vi "MainInterface_test.vi"() -> ()   [LabVIEW 2018]
uses:
  StateMachine.ctl
  System.Windows.Forms
  <vilib>/Platform/TimedLoop/XDataNode/timing_clust.ctl
  <vilib>/Platform/TimedLoop/XDataNode/nitl_modes.ctl
  <vilib>/Platform/TimedLoop/XDataNode/wakeup.ctl
  <vilib>/platform/TimedLoop/XDataNode/XDataNode.xnode
  General Libraries/Photon Filtering.lvlib
  <vilib>/Platform/TimedLoop/XDataNode/XDNodeRunTimeDep.lvlib
  Read and Save Files/RW_Protocols.lvlib
  General Libraries/myFFT.lvlib
panel:
  in  "PictureBox":refnum<k24>(container)
  out "size(s)":i32[](array[numeric])
  in  "Array":dbl[][](array[numeric])
  out "MemoryGetImageData":variant
  in  "loop state":T1
  out "x > 0?":bool
  out "result array":dbl[][](array[numeric])
  in  "saving name":string="D:\\Data\\Mai\\2019-03-19\\images NbZ=10\\noUS"
  in  "Save all raw images":bool
  in  "run statistics":bool
  in  "flush queue":bool
  in  "Flush Pile":bool
  out "Phase array":dbl[](array[numeric])
  out "sequence NbXZ":dbl[][](array[numeric])
  out "Frame Droped":bool
  in  "buffer":i32
  out "# elements in queue":i32
  in  "Stored data":cluster{dbl, dbl}[](array[cluster])=[{2.048368921229373, 0.13043478260869565}, {2.0513479056383823, 0.2608695652173913}, {2.0543268900473914, 0.043478260869565216}, {2.0573058744564006, 0.08695652173913043}, {2.0602848588654097, 0.34782608695652173}, {2.063263843274419, 0.5217391304347826}, {2.066242827683428, 0.391304347826087}, {2.069221812092437, 0.5652173913043478}, {2.072200796501446, 0.6956521739130435}, {2.0751797809104553, 0.5217391304347826}, {2.0781587653194644, 0.7391304347826086}, {2.0811377497284735, 0.5652173913043478}, {2.0841167341374827, 0.7391304347826086}, {2.087095718546492, 0.5652173913043478}, {2.090074702955501, 0.6086956521739131}, {2.09305368736451, 0.391304347826087}, {2.096032671773519, 0.43478260869565216}, {2.0990116561825283, 0.17391304347826086}, {2.1019906405915374, 0.34782608695652173}, {2.1049696250005465, 0.21739130434782608}, {2.1079486094095556, 0.13043478260869565}, {2.1109275938185648, 0.08695652173913043}, {2.113906578227574, 0.13043478260869565}]
  in  "live":bool
  in  "Tab Control":enum32{"Camera", "Trigger", "configuration"}(tab)
  in  "exposure (us)":i32(slide) caption="exposure" scale=50.0..30000000.0
  in  "gain":i32(slide) scale=32.0..2047.0
  in  "VCD Properties":bool
  in  "Period loop (ms)":i64=150
  in  "sofware triffer":bool
  in  "Trigger ON":bool
  in  "LogFile":bool
  out "error out":errorcluster
  in  "Stop Button":bool
  in  "view tab":T2(tab)
  in  "zoom factor":dbl(slide)=1.0101010101010102 scale=0.0..10.0
  in  "snap FFT":bool
  in  "ICImagingControl":refnum<k7>(container)
  out "Image":T3(plugin-control)
  out "Image Type :":T4 items=["Grayscale (U8)", "Grayscale (I16)", "Grayscale (SGL)", "Complex (CSG)", "RGB (U32)", "HSL (U32)", "RGB (U64)", "Grayscale (U16)"]
  in  "save image 2":bool
  out "data":dbl[][](array[numeric])
  in  "filtered int/phase":bool=TRUE
  in  "Filter on/off":bool=TRUE
  in  "Mask ON":bool
  out "filtered  FFT":dbl[][](graph)
  out "FFT":dbl[][](graph)
  out "value":dbl format="%#_8e"
  in  "Start time":dbl
  in  "FFT int/phase":bool=TRUE
  in  "update loop":bool
  in  "save scan":bool
  out "reconstructed image":dbl[][](graph)
  out "FFT acquire Graph":dbl[][](graph)
  in  "sequence list":i32[](listbox)
  in  "start sequence":bool
  out "N current shoot":i32
  in  "phase offset":dbl format="%#_13g"
  in  "scan name":string="D:\\Data\\Mai\\2019-03-19\\images NbZ=10\\noUS"
  in  "Current scan Tag":i32
  in  "active col":i32
  in  "statistics show":u16(ring)=2 items=["average", "variance", "S/N"]
  out "filtered  averaged":dbl[][](graph)
  out "FFT averaged":dbl[][](graph)
  in  "clear bin":bool
  in  "save noise":bool
  out "Total points num":i32
  out "current averaging":i32
  out "sequence cluster":T5
  out "fft cluster":T6
  # "Watch out more maximum queue size of 200 (update if necessary)"
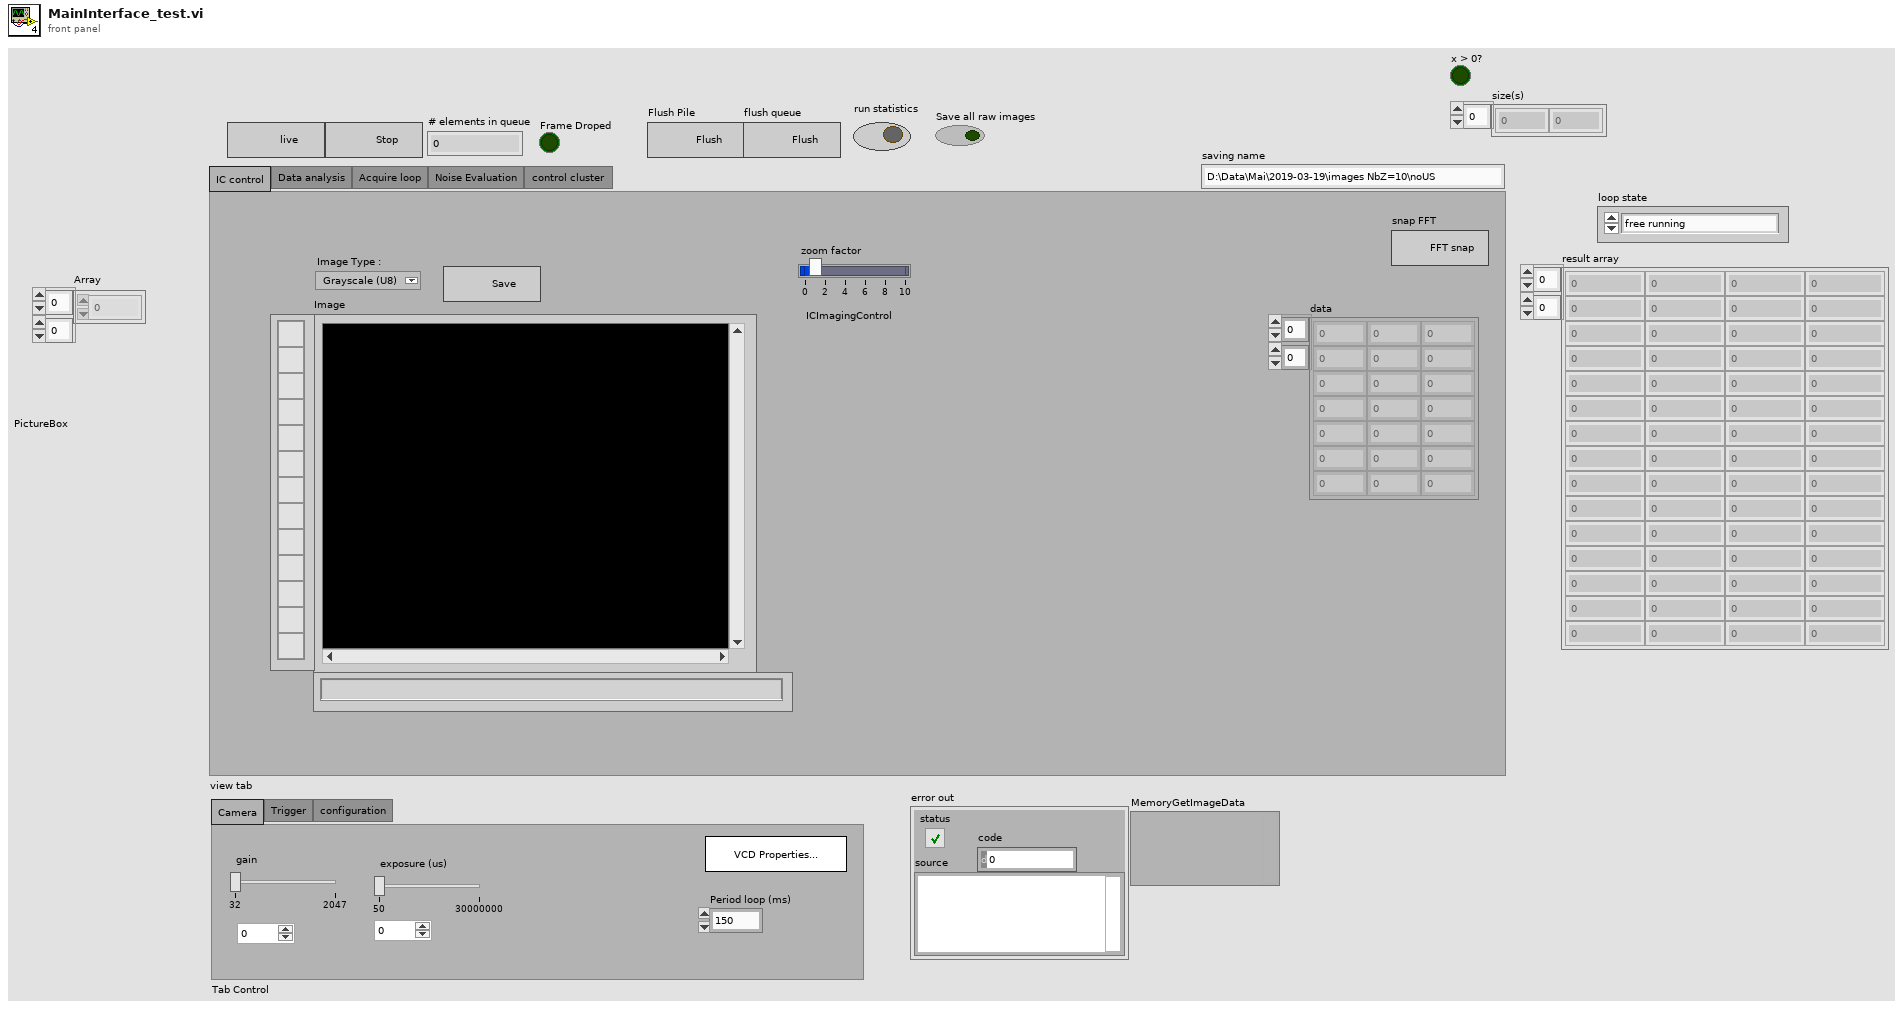
[diagram p1: front panel]
types:
  T1 = typedef "StateMachine.ctl" = enum16{"free running", "sequence recording", "run statistics"}
  T2 = enum32{"IC control", "Data analysis", "Acquire loop", "Noise Evaluation", "control cluster "}
  T3 = typedef "IMAQ Image.ctl" = refnum<image>
  T4 = typedef "Image Type" = u32
  T5 = cluster{"TypeOfSequence":string, "FreqSonde":dbl, "NbHemicycle":dbl, "Tau_cam":dbl, "DurWaveform":dbl, "Prof":dbl, "Nevent":i32, "nuX0":dbl, "nuZ0":dbl}
  T6 = cluster{"dFx":dbl, "dFy":dbl, "Nx":i32, "Ny":i32, "FxMax":dbl, "FyMax":dbl, "Xwidth":dbl, "Ywidth":dbl, "dx":dbl, "dy":dbl, "Fx points":dbl[], "X points":dbl[], "Y points":dbl[], "Fy points":dbl[]}
  T7 = enum8{"Enabled", "Disabled", "Disabled and Grayed Out"}
  T8 = cluster{"Nx fft":i32, "Fx Vector":dbl[], "Ny fft":i32, "Fy-Vector":dbl[]}
  T9 = cluster{"Image Pixels (U16)":u16[][], "Start time":dbl, "buffer":i32}
  T10 = typedef "XDNodeRunTimeDep.lvlib/timing_clust.ctl" = cluster{"Expected End [f-1]":u64, "Actual End [f-1]":u64, "Finished Late? [f-1]":bool, "Expected End [i-1]":u64, "Actual End [i-1]":u64, "Finished Late? [i-1]":bool, "Expected Start [i]":u64, "Actual Start [i]":u64, "Expected Start [f]":u64, "Actual Start [f]":u64, "Source Name":string, "Structure Name":string, "Period":i64, "Deadline":i64, "Offset":i64, "Start":i64, "Priority":i32, "Timeout":i32, "Mode":T11, "Wakeup Reason":T12, "Error":errorcluster, "Source Type":string, "Secondary Source Type":string, "Global End Time":u64, "Global Start Time":u64, "Frame Duration":u64, "Iteration Duration":u64, "Assigned CPU":i32, "I/O Scan Engine Mode":u32}
  T11 = typedef "XDNodeRunTimeDep.lvlib/nitl_modes.ctl" = enum32{"No Change", "Process missed periods, maintain original phase", "Discard missed periods, maintain original phase", "Process missed periods, ignore original phase", "Discard missed periods, ignore original phase"}
  T12 = typedef "XDNodeRunTimeDep.lvlib/wakeup.ctl" = enum32{"Normal", "Aborted", "Asynchronous wakeup", "Timing source error", "Timed loop error", "Timeout"}
  T13 = enum16{"Brightness", "Color Enable", "Contrast", "Exposure", "Focus", "Gain", "Gamma", "Hue", "Iris", "Pan", "Roll", "Saturation", "Sharpness", "Tilt", "Whitebalance", "Zoom", "Whitebalance Blue", "Whitebalance Red"}
  T14 = cluster{"Rows Per Strip":i32, "Photometric":i32, "Compression Type":i32}
  T15 = cluster{"Image Pixels (U16)":u16[][], "SampleStartTime":dbl, "Index":i32}
  T16 = cluster{"Filter on/off":bool, "filtered int/phase":bool, "Mask ON":bool, "FFT int/phase":bool}
  T17 = cluster{"tagged photons":dbl[][], "FFT modulous":dbl[][]}
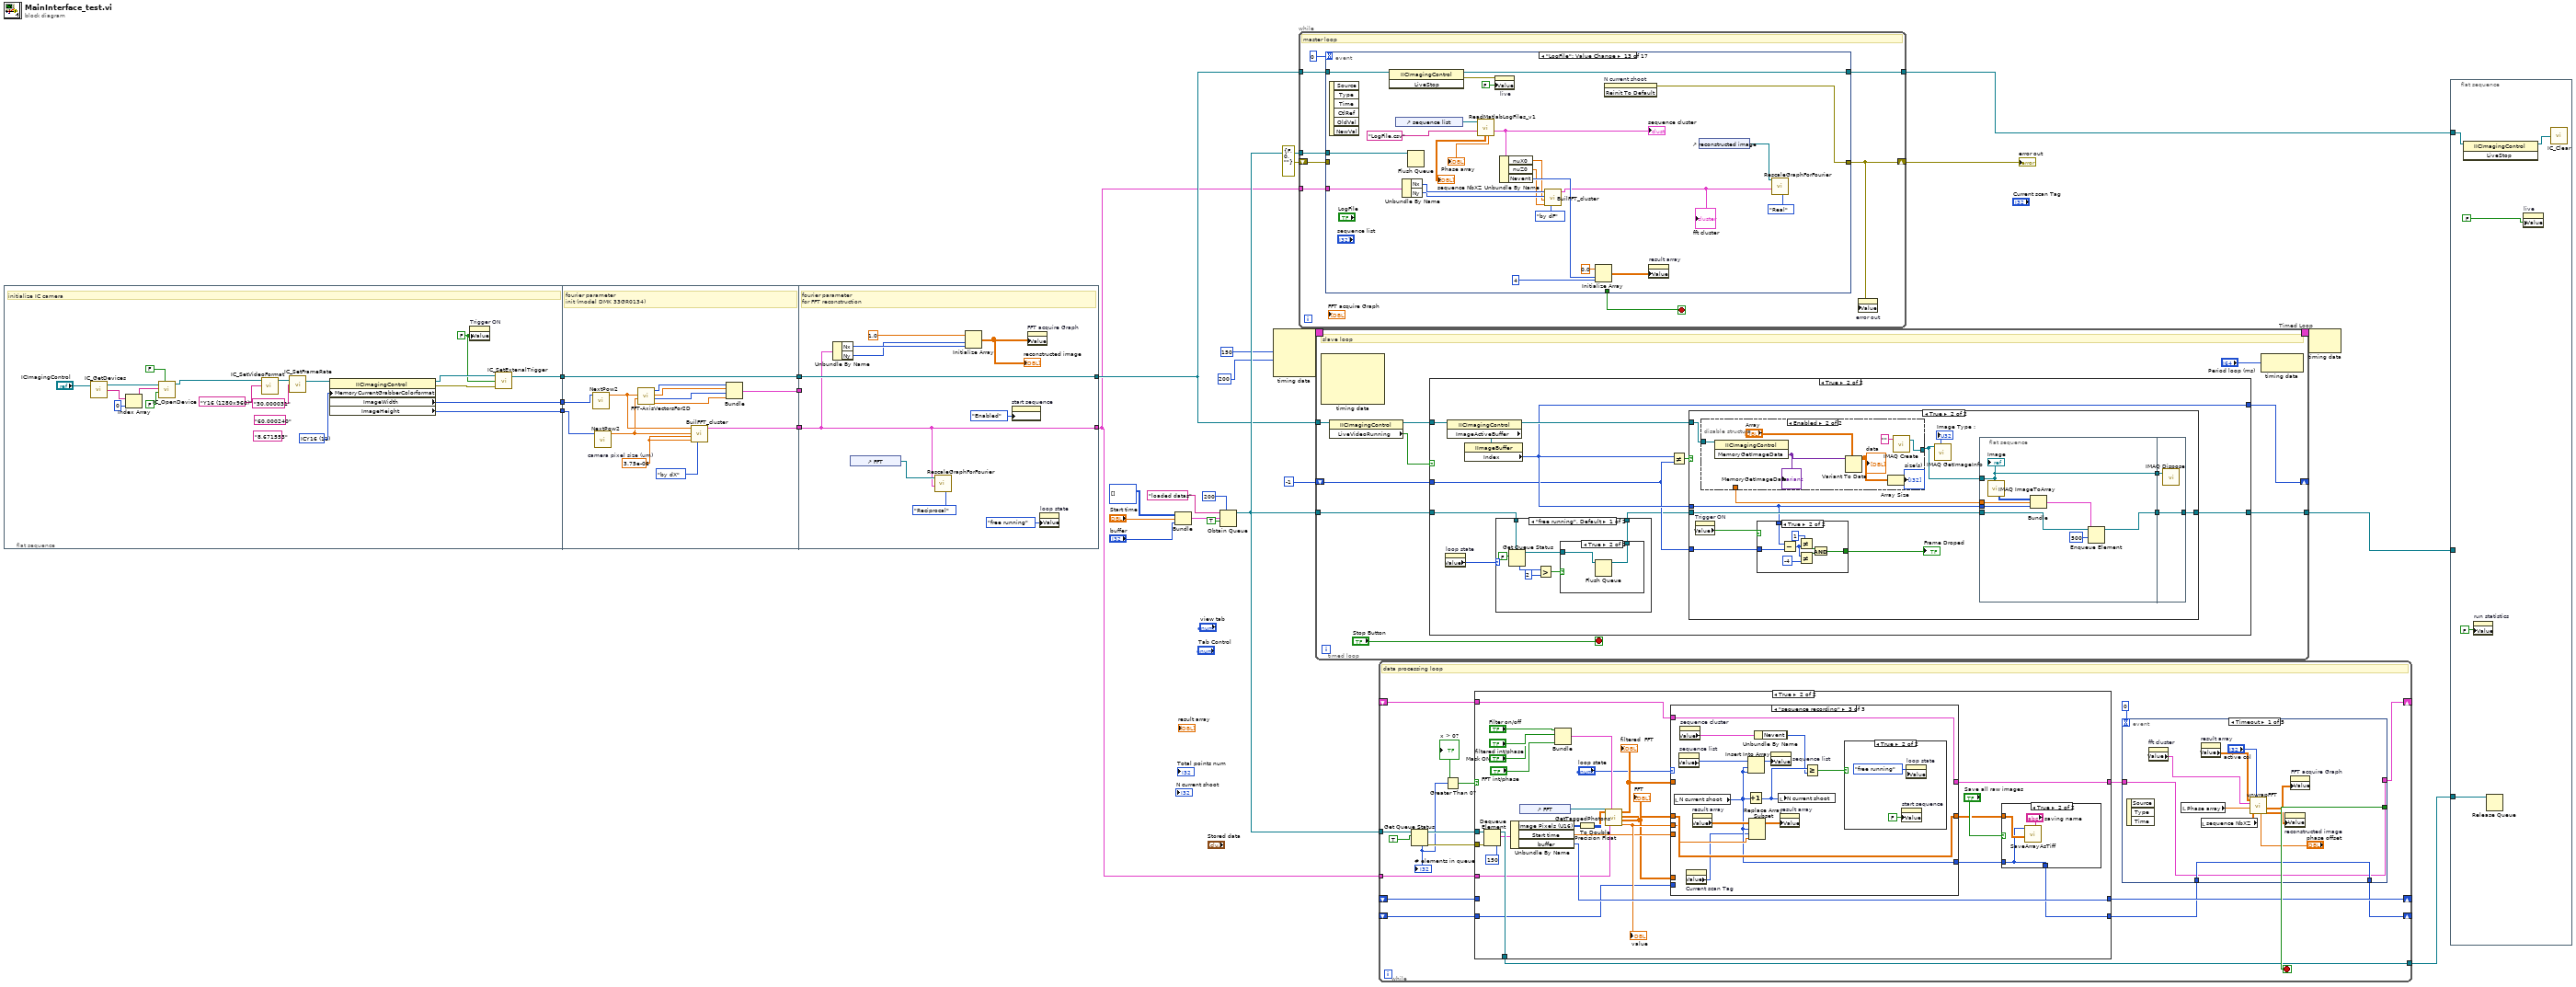
[diagram p0: block diagram]
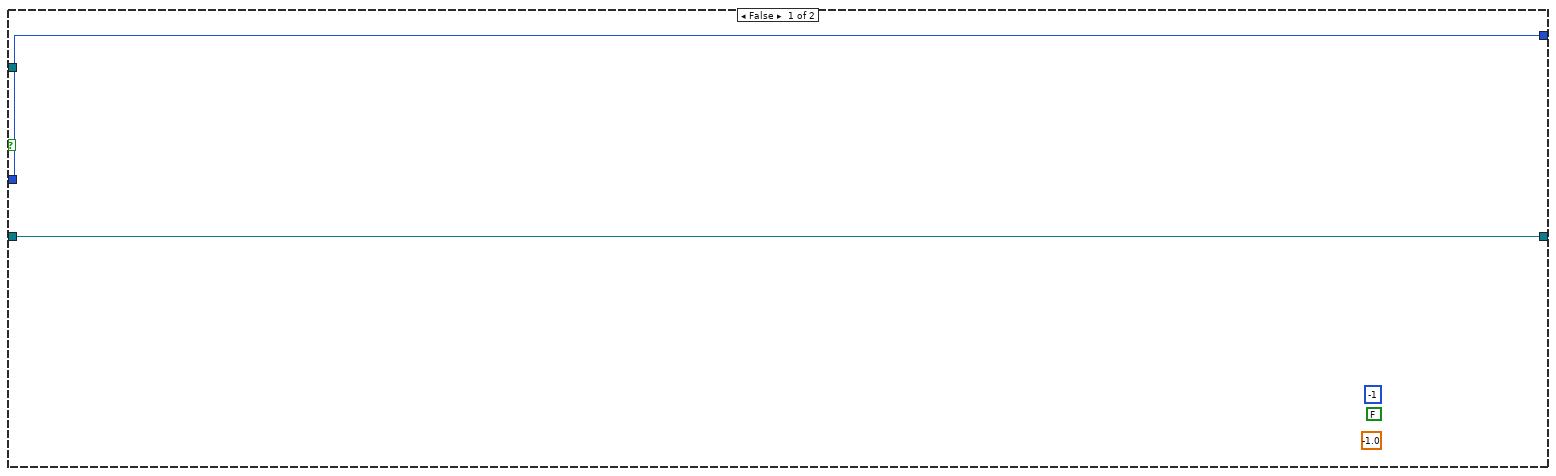
[diagram p2: hidden frame]
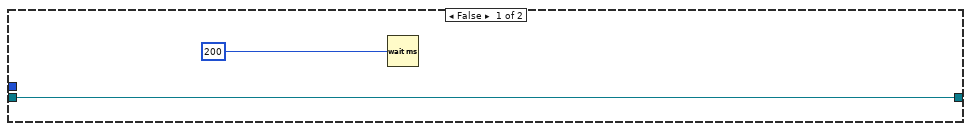
[diagram p5: hidden frame]
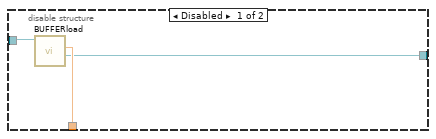
[diagram p6: hidden frame]
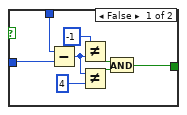
[diagram p7: hidden frame]
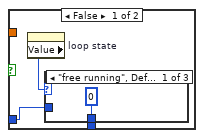
[diagram p9: hidden frame]
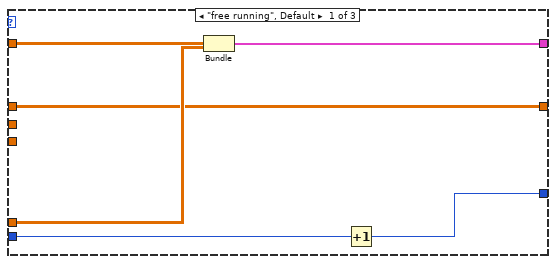
[diagram p12: hidden frame]
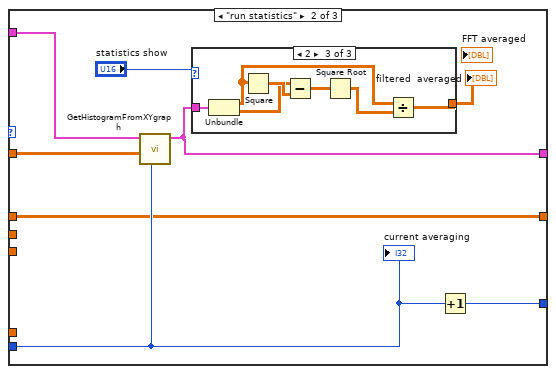
[diagram p13: hidden frame]
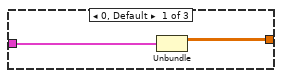
[diagram p14: hidden frame]
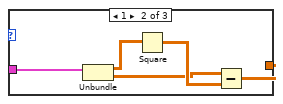
[diagram p15: hidden frame]
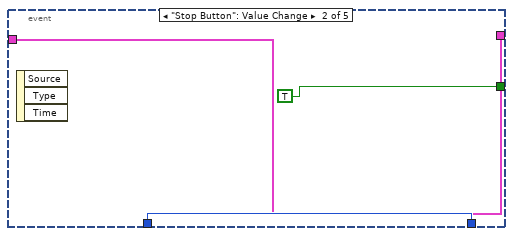
[diagram p17: hidden frame]
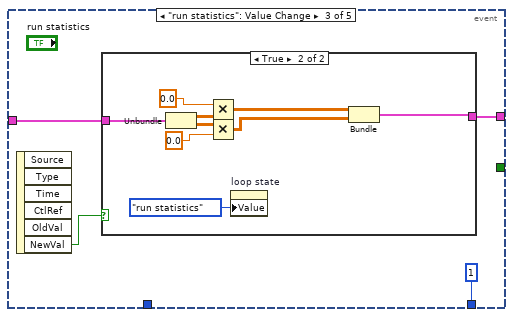
[diagram p18: hidden frame]
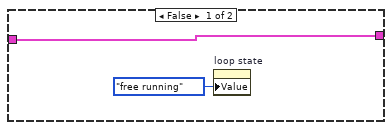
[diagram p19: hidden frame]
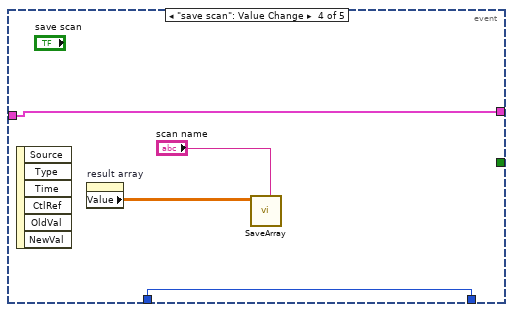
[diagram p20: hidden frame]
diagram:
  n1 = flat-sequence {
    tunnel: [w30] -> w9
    tunnel: [w28] -> w8
    tunnel: [w27] -> w7
    tunnel: w9 -> [w58]
    tunnel: w8 -> [w57]
    tunnel: w7 -> [w56]
    tunnel: [w58] -> w6
    tunnel: [w51] -> w5
    tunnel: [w47] -> w3
    tunnel: [w68] -> w20
    tunnel: w6 -> [w68]
    tunnel: w5 -> [_]
    tunnel: [w60] -> w2
    tunnel: w3 -> [w60]
    frame #0 {
      w31 = FALSE ("Trigger ON")
      (unwired) "8,671553"
      (unwired) "60,000240" ("FrameRate")
      w35 = 11 items=["ICRGB32"=1, "ICRGB24"=2, "ICRGB565"=3, "ICRGB555"=4, "ICY8"=5, "ICUYVY"=6, "ICY800"=7, "ICYGB1"=8, "ICYGB0"=9, "ICBY8"=10, "ICY16"=11] ("MemoryCurrentGrabberColorformat")
      # "initialize IC camera"
      n2 = call <userlib>:"IC_GetDevices.vi"("ICImagingControl In"="ICImagingControl") -> ("ICImagingControl Out"=w42:refnum<k7>, "Devices"=w44:string[])  [unwired: 1 in, 1 out]
      n3 = Index Array(array=w44, index=0) -> (element=w41:string)
      n4 = call <userlib>:"IC_OpenDevice.vi"("Color"=FALSE, "Live"=FALSE, "Device"=w41, "ICImagingControl In"=w42) -> ("ICImagingControl Out"=w38:refnum<k7>)  [unwired: 2 in, 5 out]
      n5 = call <userlib>:"IC_SetVideoFormat.vi"("VideoFormat"="Y16 (1280x960)", "ICImagingControl In"=w38) -> ("ICImagingControl Out"=w37:refnum<k7>)  [unwired: 1 in, 2 out]
      n6 = call <userlib>:"IC_SetFrameRate.vi"("FrameRate"="30,000031", "ICImagingControl In"=w37) -> ("ICImagingControl Out"=w36:refnum<k7>)  [unwired: 1 in, 1 out]
      n7 = property class="IICImagingControl"(reference=w36, "MemoryCurrentGrabberColorformat"=w35) -> (reference out=w32:refnum<k7>, error out=w29:errorcluster, "ImageWidth"=w28:i32, "ImageHeight"=w27:i32)  [unwired: 1 in]
      n8 = property on="Trigger ON" class="Bool (strict)"("Value"=w31) -> ()  [unwired: 2 in, 2 out]
      n9 = call <userlib>:"IC_SetExtenalTrigger.vi"("Error In (no error)"=w29, "Trigger"=w31, "ICImagingControl In"=w32) -> ("ICImagingControl Out"=w30:refnum<k7>)  [unwired: 1 out]
    }
    frame #1 {
      w48 = 3.75e-06  # camera pixel size (um)
      # "fourier parameter\ninit (model DMK 33GR0134)"
      n10 = call "NextPow2.vi"("x"=w57) -> ("2^x"=w50:dbl)  [unwired: 10 in]
      n11 = call "NextPow2.vi"("x"=w56) -> ("2^x"=w49:dbl)  [unwired: 10 in]
      n12 = call "FFT-AxisVectorsFor2D.vi"("Ny in"=w49, "Nx in"=w50) -> ("Fy-Vector"=w52:dbl[], "Ny fft"=w53:i32, "Fx Vector"=w54:dbl[], "Nx fft"=w55:i32)  [unwired: 6 in]
      n13 = call "BuilFFT_cluster.vi"("Enum"=enum16{"by dF", "by dX"}."by dX", "input Y"=w48, "input X"=w48, "Ny"=w49, "Nx"=w50) -> ("fft cluster"=w47:T6)  [unwired: 6 in]
      n14 = Bundle("Nx fft"=w55, "Fx Vector"=w54, "Ny fft"=w53, "Fy-Vector"=w52) -> (w51:T8)  [unwired: 1 in]
    }
    frame #2 {
      # "fourier parameter\nfor FFT reconstruction"
      n15 = Unbundle By Name(w60) -> ("Nx"=w66:i32, "Ny"=w65:i32)
      n16 = control-ref of="FFT"() -> (w62:refnum<vi>)
      n17 = call "RescaleGraphForFourier.vi"("fft reference"=w62, "fft cluster"=w60, "Enum"=enum16{"Reciprocal", "Real"}."Reciprocal") -> ()  [unwired: 8 in]
      n18 = Initialize Array(1.0 ("r"), w65, w66) -> (w64:dbl[][])
      "reconstructed image" <- w64
      n19 = property on="start sequence" class="Bool (strict)"("DisabledEnum"=T7."Enabled" ("Disabled")) -> ()  [unwired: 2 in, 2 out]
      n20 = property on="FFT acquire Graph" class="IntGraph (strict)"("Value"=w64) -> ()  [unwired: 2 in, 2 out]
      n21 = property on="loop state" class="Enum (strict)"("Value"=StateMachine."free running" ("loop state")) -> ()  [unwired: 2 in, 2 out]
    }
  }
  n22 = Bundle("Image Pixels (U16)"=u16[][] [], "Start time"="Start time", "buffer"="buffer") -> (w23:T9)  [unwired: 1 in]
  n23 = Obtain Queue(max queue size (-1, unlimited)=200, name (unnamed)="loaded datas", element data type=w23, create if not found? (T)=TRUE) -> (queue out=w22:refnum<queue>)  [unwired: 1 in, 2 out]
  n24 = node-c288(i64 150 ("Period"), 200 ("Priority")) -> (w15:T10)  [unwired: 2 in]
  n25 = while {
    tunnel: w20 -> [w75]
    tunnel: [w76] -> w16
    shift-right: [w70] -> w17
    shift-left: errorcluster {"status"=FALSE, "code"=0, "source"=""} ("error out") -> [w74]
    tunnel: w22 -> [w73]
    tunnel: w2 -> [w69]
    stop <- w72 stop-if-true
    # "master loop"
    n26 = event shown="[12] \"LogFile\": Value Change" {
      selector: _ -> [_ _ _ _ _ _ _ _ _ _ _ _ _ _ _ _ _]
      dyn-events: _ -> [_ _ _ _ _ _ _ _ _ _ _ _ _ _ _ _ _]
      timeout: 0 -> [_ _ _ _ _ _ _ _ _ _ _ _ _ _ _ _ _]
      tunnel: [_ TRUE _ _ _ _ _ _ _ _ _ _ _ _ _ _ _] -> w72
      tunnel: [w77 w80 _ w84 w86 w97 w102 w105 _ w114 _ w128 w152 w158 w171 w182 w192] -> w76
      tunnel: w75 -> [w77 w80 _ w85 w87 w94 w103 w104 _ w115 w123 w129 w153 w157 w175 w183 w193]
      tunnel: [w78 w79 _ _ w88 w96 w100 w106 _ w113 w125 _ w145 _ _ _ w191] -> w70
      tunnel: w74 -> [w78 w79 w82 _ w88 w95 w101 w107 _ w112 _ _ _ _ _ _ w191]
      tunnel: w73 -> [_ _ w83 _ _ _ _ _ w110 _ _ _ w149 _ _ _ _]
      tunnel: w69 -> [_ _ _ _ _ _ _ _ _ _ _ _ w143 _ _ _ _]
      event Timeout {
        n27 = event-data() -> ()  [unwired: 1 in, 3 out]
      }
      event "Stop Button": Value Change {
        n28 = event-data() -> ()  [unwired: 1 in, 6 out]
      }
      event "flush queue": Value Change {
        n29 = event-data() -> ()  [unwired: 1 in, 6 out]
        n30 = Flush Queue(queue=w83, error in (no error)=w82) -> ()  [unwired: 3 out]
      }
      event "VCD Properties": Value Change {
        n31 = event-data() -> ()  [unwired: 1 in, 6 out]
        n32 = invoke class="IICImagingControl" method="ShowPropertyDialog"(reference=w85) -> (reference out=w84:refnum<k7>)  [unwired: 2 in, 2 out]
      }
      event "live": Value Change {
        n33 = event-data() -> ("NewVal"=w89:bool)  [unwired: 1 in, 5 out]
        n34 = case shown="False" w89 {
          tunnel: w87 -> [w91 w93]
          tunnel: [w90 w92] -> w86
          frame False {
            n35 = invoke class="IICImagingControl" method="LiveStop"(reference=w91) -> (reference out=w90:refnum<k7>)  [unwired: 2 in, 2 out]
          }
          frame True {
            n36 = call <userlib>:"IC_LiveStart.vi"("ICImagingControl 3"=w93) -> ("ICImagingControl 2"=w92:refnum<k7>)
          }
        }
      }
      event "zoom factor": Value Change {
        n37 = event-data() -> ()  [unwired: 1 in, 6 out]
        n38 = property class="IICImagingControl" props=["ZoomRange"](reference=w94, error in=w95) -> (reference out=w97:refnum<k7>, error out=w96:errorcluster)  [unwired: 1 out]
      }
      event "exposure (us)": Value Change {
        n39 = event-data() -> ()  [unwired: 1 in, 6 out]
        n40 = call <userlib>:"IC_SetPropertyValue.vi"("Error In (no error)"=w101, "Value"="exposure (us)", "Property"=T13."Exposure", "ICImagingControl In"=w103) -> ("Error Out"=w100:errorcluster, "ICImagingControl Out"=w102:refnum<k7>)
      }
      event "gain": Value Change {
        n41 = event-data() -> ()  [unwired: 1 in, 6 out]
        n42 = call <userlib>:"IC_SetPropertyValue.vi"("Error In (no error)"=w107, "Value"="gain", "Property"=T13."Gain", "ICImagingControl In"=w104) -> ("Error Out"=w106:errorcluster, "ICImagingControl Out"=w105:refnum<k7>)
      }
      event "Flush Pile": Value Change {
        n43 = event-data() -> ()  [unwired: 1 in, 6 out]
        n44 = Flush Queue(queue=w110) -> ()  [unwired: 1 in, 3 out]
      }
      event "Trigger ON": Value Change {
        n45 = event-data() -> ("NewVal"=w111:bool)  [unwired: 1 in, 5 out]
        n46 = call <userlib>:"IC_SetExtenalTrigger.vi"("Error In (no error)"=w112, "Trigger"=w111, "ICImagingControl In"=w115) -> ("Error Out"=w113:errorcluster, "ICImagingControl Out"=w114:refnum<k7>)
      }
      event "save image 2": Value Change {
        n47 = event-data() -> ()  [unwired: 1 in, 6 out]
        n48 = invoke class="IICImagingControl" method="LiveStop"(reference=w123) -> (reference out=w122:refnum<k7>)  [unwired: 2 in, 2 out]
        n49 = property class="IICImagingControl" props=["ImageActiveBuffer"](reference=w122) -> (reference out=w119:refnum<k7>)  [unwired: 1 in, 2 out]
        n50 = property on="saving name" class="Str"() -> ("Value"=w117:string)  [unwired: 2 in, 2 out]
        n51 = call "FetchTargetFile.vi"("Use default Folder"=TRUE, "FileName"=w117) -> ("Full File Path"=w116:path)  [unwired: 9 in]
        n52 = call "BUFFERload.vi"("ICImagingControl In"=w119) -> ("Image Out"=w120:T3)  [unwired: 6 in, 4 out]
        n53 = call-poly "IMAQ Write File 2"("TIFF Options"=T14 {"Rows Per Strip"=0, "Photometric"=1, "Compression Type"=0}, "File Path"=w116, "Image"=w120) -> ("error out"=w126:errorcluster, "Image Out (duplicate)"=w121:T3)  [unwired: 7 in]
        n54 = call "IMAQ Dispose"("Image"=w121, "error in (no error)"=w126) -> ("error out"=w125:errorcluster)  [unwired: 4 in]
      }
      event "snap FFT": Value Change {
        n55 = event-data() -> ()  [unwired: 1 in, 6 out]
        n56 = invoke class="IICImagingControl" method="LiveStop"(reference=w129) -> (reference out=w131:refnum<k7>)  [unwired: 2 in, 2 out]
        n57 = property class="IICImagingControl" props=["ImageActiveBuffer"](reference=w131) -> (reference out=w130:refnum<k7>)  [unwired: 1 in, 2 out]
        n58 = call <userlib>:"IC_ActiveBuffer_to_IMAQ.vi"("ICImagingControl In"=w130) -> ("ICImagingControl Out"=w128:refnum<k7>, "Image Out"=w127:T3)  [unwired: 2 in, 2 out]
        n59 = call "IMAQ ImageToArray"("Image"=w127) -> ()  [unwired: 3 in, 5 out]
        n60 = call "IMAQ Dispose"() -> ()  [unwired: 6 in, 1 out]
      }
      event "LogFile": Value Change {
        n61 = event-data() -> ()  [unwired: 1 in, 6 out]
        n62 = invoke class="IICImagingControl" method="LiveStop"(reference=w153) -> (reference out=w152:refnum<k7>, error out=w151:errorcluster)  [unwired: 2 in, 1 out]
        n63 = control-ref of="sequence list"() -> (w155:refnum<vi>)
        n64 = Unbundle By Name(w143) -> ("Nx"=w141:i32, "Ny"=w140:i32)
        n65 = Flush Queue(queue=w149) -> ()  [unwired: 1 in, 3 out]
        n66 = call "ReadMatlabLogFiles_v1.vi"("FileName"="LogFile.csv" ("FileName For Matlab load"), "sequence list REF"=w155) -> ("sequence cluster"=w148:T5, "Phase array unit"=→"Phase array":dbl[], "all values"=→"sequence NbXZ":dbl[][])  [unwired: 4 in, 3 out]
        "sequence cluster" <- w148
        n67 = property on="live" class="Bool (strict)"(error in=w151, "Value"=FALSE ("live")) -> ()  [unwired: 1 in, 2 out]
        n68 = Unbundle By Name(w148) -> ("nuX0"=w139:dbl, "nuZ0"=w138:dbl, "Nevent"=w147:i32)
        n69 = call "BuilFFT_cluster.vi"("Enum"=enum16{"by dF", "by dX"}."by dF", "input Y"=w138, "input X"=w139, "Ny"=w140, "Nx"=w141) -> ("fft cluster"=w137:T6)  [unwired: 6 in]
        "fft cluster" <- w137
        n70 = Initialize Array(0.0 ("element"), w147, 4 ("dimension size")) -> (w133:dbl[][])
        n71 = invoke on="N current shoot" class="DigNum (strict)" method="Reinit To Default"() -> (error out=w145:errorcluster)  [unwired: 3 in, 2 out]
        n72 = property on="result array" class="Arr (strict)"("Value"=w133) -> ()  [unwired: 2 in, 2 out]
        n73 = control-ref of="reconstructed image"() -> (w136:refnum<vi>)
        n74 = call "RescaleGraphForFourier.vi"("fft reference"=w136, "fft cluster"=w137, "Enum"=enum16{"Reciprocal", "Real"}."Real") -> ()  [unwired: 8 in]
      }
      event "start sequence": Value Change {
        n75 = event-data() -> ("NewVal"=w156:bool)  [unwired: 1 in, 5 out]
        n76 = case shown="True" w156 {
          tunnel: [w162 w167] -> w158
          tunnel: w157 -> [w163 w166]
          frame False {
            n77 = invoke class="IICImagingControl" method="LiveStop"(reference=w163) -> (reference out=w162:refnum<k7>, error out=w161:errorcluster)  [unwired: 2 in, 1 out]
            n78 = property on="live" class="Bool (strict)"(error in=w161, "Value"=FALSE ("live")) -> ()  [unwired: 1 in, 2 out]
            n79 = property on="loop state" class="Enum (strict)"("Value"=StateMachine."free running" ("loop state")) -> ()  [unwired: 2 in, 2 out]
          }
          frame True {
            n80 = flat-sequence {
              tunnel: w166 -> [w168]
              tunnel: [w168] -> w165
              frame #0 {
                n81 = Wait (ms)(milliseconds to wait=u32 10) -> ()  [unwired: 1 out]
                n82 = property on="loop state" class="Enum (strict)"("Value"=StateMachine."sequence recording" ("loop state")) -> ()  [unwired: 2 in, 2 out]
              }
            }
            n83 = invoke class="IICImagingControl" method="LiveStart"(reference=w165) -> (reference out=w167:refnum<k7>)  [unwired: 2 in, 2 out]
            n84 = property on="live" class="Bool (strict)"("Value"=TRUE ("live")) -> ()  [unwired: 2 in, 2 out]
          }
        }
      }
      event "update loop": Value Change {
        n85 = event-data() -> ()  [unwired: 1 in, 6 out]
        n86 = invoke class="IICImagingControl" method="LiveStop"(reference=w175) -> (reference out=w172:refnum<k7>, error out=w173:errorcluster)  [unwired: 2 in, 1 out]
        n87 = property on="live" class="Bool (strict)"(error in=w173, "Value"=FALSE ("live")) -> ()  [unwired: 1 in, 2 out]
        n88 = flat-sequence {
          tunnel: w172 -> [w180]
          tunnel: [w180] -> w171
          frame #0 {
            n89 = property on="Current scan Tag" class="DigNum (strict)"() -> ("Value"=w178:i32)  [unwired: 2 in, 2 out]
            n90 = property on="sequence list" class="MCListbox (strict)"("Value"=i32[] []) -> ()  [unwired: 2 in, 2 out]
            n91 = Increment(x=w178) -> (x+1=w177:i32)
            n92 = property on="N current shoot" class="DigNum (strict)"("Value"=0 ("N current shoot")) -> ()  [unwired: 2 in, 2 out]
            n93 = property on="Current scan Tag" class="DigNum (strict)"("Value"=w177) -> ()  [unwired: 2 in, 2 out]
          }
        }
      }
      event "clear bin": Value Change {
        n94 = event-data() -> ()  [unwired: 1 in, 6 out]
        n95 = property on="live" class="Bool (strict)"() -> ("Value"=w181:bool)  [unwired: 2 in, 2 out]
        n96 = case shown="True" w181 {
          tunnel: w183 -> [w184 w190]
          tunnel: [w184 w188] -> w182
          frame False {
          }
          frame True {
            n97 = invoke class="IICImagingControl" method="LiveStop"(reference=w190) -> (reference out=w189:refnum<k7>)  [unwired: 2 in, 2 out]
            n98 = property on="Total points num" class="DigNum (strict)"("Value"=0 ("Total points num")) -> (error out=w185:errorcluster)  [unwired: 2 in, 1 out]
            n99 = invoke on="Total points num" class="DigNum (strict)" method="Reinit To Default"(error in=w185) -> (error out=w187:errorcluster)  [unwired: 2 in, 2 out]
            n100 = invoke class="IICImagingControl" method="LiveStart"(reference=w189, error in=w187) -> (reference out=w188:refnum<k7>)  [unwired: 1 in, 2 out]
          }
        }
      }
      event "sofware triffer": Value Change {
        n101 = event-data() -> ()  [unwired: 1 in, 6 out]
        n102 = call <userlib>:"IC_SoftwareTrigger.vi"("ICImagingControl 3"=w193) -> ("ICImagingControl 2"=w192:refnum<k7>)
      }
    }
    n103 = property on="error out" class="Clust (strict)"("Value"=w70) -> ()  [unwired: 2 in, 2 out]
  }
  "error out" <- w17
  n104 = timed-loop "Timed Loop" {
    tunnel: w20 -> [w201]
    shift-right: [w198] -> _
    shift-left: -1 ("Index") -> [w202]
    tunnel: w22 -> [w197]
    tunnel: [w196] -> w19
    timing: w15 -> [_]
    timing-out: [_] -> w14
    stop <- "Stop Button" stop-if-true
    # "slave loop"
    n105 = node-c288() -> ()  [unwired: 1 in, 5 out]
    n106 = property class="IICImagingControl"(reference=w201) -> (reference out=w200:refnum<k7>, "LiveVideoRunning"=w199:bool)  [unwired: 1 in, 1 out]
    n107 = case shown="True" w199 {
      tunnel: w202 -> [w208 w212]
      tunnel: w200 -> [_ w218]
      tunnel: [w208 w213] -> w198
      tunnel: w197 -> [w207 w211]
      tunnel: [w207 w214] -> w196
      frame False {
        (unwired) -1.0 ("SampleStartTime")
        (unwired) FALSE
        (unwired) -1 ("Index")
      }
      frame True {
        n108 = property on="loop state" class="Enum (strict)"() -> ("Value"=w209:T1)  [unwired: 2 in, 2 out]
        n109 = property class="IICImagingControl"(reference=w218) -> (reference out=w216:refnum<k7>, "ImageActiveBuffer"=w217:refnum<k7>)  [unwired: 1 in, 1 out]
        n110 = property class="IImageBuffer"(reference=w217) -> ("Index"=w213:i32)  [unwired: 1 in, 2 out]
        n111 = case shown="\"free running\", Default" w209 {
          tunnel: w211 -> [w225 w229]
          tunnel: [w220 w229] -> w210
          frame "free running", Default {
            n112 = Get Queue Status(queue=w225, return elements? (F)=FALSE) -> (queue out=w221:refnum<queue>, # elements in queue=w224:i32)  [unwired: 1 in, 6 out]
            n113 = Greater?(x=w224, y=2) -> (0:w222:bool)
            n114 = case shown="True" w222 {
              tunnel: w221 -> [w226 w228]
              tunnel: [w226 w227] -> w220
              frame False {
              }
              frame True {
                n115 = Flush Queue(queue=w228) -> (queue out=w227:refnum<queue>)  [unwired: 1 in, 2 out]
              }
            }
          }
          frame "sequence recording" {
          }
        }
        n116 = Not Equal?(x=w213, y=w212) -> (x != y?=w215:bool)
        n117 = case shown="True" w215 {
          tunnel: w216 -> [_ w243]
          tunnel: w210 -> [w230 w242]
          tunnel: [w230 w241] -> w214
          tunnel: w213 -> [_ w234]
          tunnel: w212 -> [_ w235]
          frame False {
            n118 = Wait (ms)(milliseconds to wait=u32 200) -> ()  [unwired: 1 out]
          }
          frame True {
            n119 = property on="Trigger ON" class="Bool (strict)"() -> ("Value"=w232:bool)  [unwired: 2 in, 2 out]
            n120 = disable-structure shown="Enabled" {
              disable-tunnel: w243 -> [w246 w253]
              disable-tunnel: [w245 _] -> w240
              disable-tunnel: [w244 w252] -> w239
              frame Disabled {
                n121 = call "BUFFERload.vi"("ICImagingControl In"=w246) -> ("Image Out"=w244:T3, "SampleStartTime"=w245:dbl)  [unwired: 6 in, 3 out]
              }
              frame Enabled {
                n122 = invoke class="IICImagingControl" method="MemoryGetImageData"(reference=w253) -> ("MemoryGetImageData"=w249:variant)  [unwired: 2 in, 2 out]
                "MemoryGetImageData" <- w249
                n123 = Variant To Data(type="Array", Variant=w249) -> (data=w248:dbl[][])  [unwired: 1 in, 1 out]
                "data" <- w248
                n124 = Array Size(array=w248) -> (size(s)=→"size(s)":i32[])
                n125 = call "IMAQ Create"("Image Name"="") -> ("New Image"=w252:T3)  [unwired: 4 in, 1 out]
              }
            }
            n126 = case shown="True" w232 {
              tunnel: w235 -> [w257 w266]
              tunnel: w234 -> [w256 w265]
              tunnel: [w255 w262] -> w233
              frame False {
                n127 = Subtract(x=w256, y=w257) -> (x-y=w261:i32)
                n128 = Not Equal?(x=-1, y=w261) -> (x != y?=w259:bool)
                n129 = Not Equal?(x=w261, y=4) -> (x != y?=w258:bool)
                n130 = And(x=w259, y=w258) -> (x .and. y?=w255:bool)
              }
              frame True {
                n131 = Subtract(x=w265, y=w266) -> (x-y=w268:i32)
                n132 = Not Equal?(x=1, y=w268) -> (x != y?=w264:bool)
                n133 = Not Equal?(x=w268, y=-4) -> (x != y?=w263:bool)
                n134 = And(x=w264, y=w263) -> (x .and. y?=w262:bool)
              }
            }
            "Frame Droped" <- w233
            n135 = call "IMAQ GetImageInfo"("Image"=w239) -> ("Image Type"=→"Image Type :":T4)  [unwired: 3 in, 7 out]
            n136 = flat-sequence {
              tunnel: w239 -> [w274]
              tunnel: [w274] -> w237
              tunnel: w242 -> [w277]
              tunnel: [w276] -> w236
              tunnel: w240 -> [w275]
              tunnel: w234 -> [w271]
              tunnel: w237 -> [w278]
              tunnel: w236 -> [w279]
              tunnel: [w279] -> w241
              frame #0 {
                n137 = call "IMAQ ImageToArray"("Image"=w274) -> ("Image Pixels (U16)"=w270:u16[][])  [unwired: 3 in, 4 out]
                n138 = Bundle("Image Pixels (U16)"=w270, "SampleStartTime"=w275, "Index"=w271) -> (w273:T15)  [unwired: 1 in]
                n139 = Enqueue Element(queue=w277, element=w273, timeout in ms (-1)=500) -> (queue out=w276:refnum<queue>)  [unwired: 1 in, 2 out]
                "Image" <- w274
              }
              frame #1 {
                n140 = call "IMAQ Dispose"("Image"=w278) -> ()  [unwired: 5 in, 1 out]
              }
            }
          }
        }
      }
    }
    n141 = node-c288("Period loop (ms)") -> ()  [unwired: 1 out]
  }
  n142 = while {
    tunnel: w22 -> [w295]
    tunnel: [w294] -> w18
    shift-right: [w288] -> _
    shift-left: _ -> [w287]
    tunnel: w2 -> [w286]
    shift-right: [w285] -> _
    shift-left: _ -> [w284]
    shift-right: [w281] -> _
    shift-left: _ -> [w280]
    stop <- w297 stop-if-true
    # "data processing loop"
    n143 = Get Queue Status(queue=w295, return elements? (F)=TRUE) -> (queue out=w293:refnum<queue>, error out=w292:errorcluster, # elements in queue=w290:i32)  [unwired: 1 in, 5 out]
    "# elements in queue" <- w290
    n144 = Greater Than 0?(x=w290) -> (x > 0?=w289:bool)
    "x > 0?" <- w289
    n145 = case shown="True" w289 {
      tunnel: [w301 w324] -> w294
      tunnel: w293 -> [w301 w326]
      tunnel: w292 -> [_ w325]
      tunnel: [w300 w323] -> w288
      tunnel: w287 -> [w300 _]
      tunnel: w286 -> [_ w319]
      tunnel: w284 -> [w299 w310]
      tunnel: [w299 w302] -> w283
      tunnel: [w298 w309] -> w282
      tunnel: w280 -> [w298 w308]
      frame False {
      }
      frame True {
        n146 = Dequeue Element(queue=w326, timeout in ms (-1)=150, error in (no error)=w325) -> (queue out=w324:refnum<queue>, element=w320:T9)  [unwired: 2 out]
        n147 = Unbundle By Name(w320) -> ("Image Pixels (U16)"=w328:u16[][], "Start time"=w321:dbl, "buffer"=w323:i32)
        n148 = control-ref of="FFT"() -> (w327:refnum<vi>)
        n149 = Bundle("Filter on/off"="Filter on/off", "filtered int/phase"="filtered int/phase", "Mask ON"="Mask ON", "FFT int/phase"="FFT int/phase") -> (w314:T16)  [unwired: 1 in]
        n150 = To Double Precision Float(number=w328) -> (double precision float=w307:dbl[][])
        n151 = call "GetTaggedPhotons.vi"("screen status"=w314, "fft cluster"=w319, "FFT reference"=w327, "double precision float"=w307) -> ("FFT full energy"=w322:dbl, "FFT modulous"=w313:dbl[][], "unfiltered image"=w306:dbl[][], "tagged photons"=w312:dbl[][])  [unwired: 4 in]
        "filtered  FFT" <- w312
        "FFT" <- w313
        "value" <- w322
        n152 = case shown="\"sequence recording\"" "loop state" {
          tunnel: w322 -> [_ _ w371]
          tunnel: w321 -> [_ _ _]
          tunnel: w312 -> [w342 w350 _]
          tunnel: w313 -> [w343 _ _]
          tunnel: w310 -> [w340 w352 _]
          tunnel: [w339 w346 w368] -> w303
          tunnel: [w344 w349 w373] -> w309
          tunnel: w308 -> [_ w351 w373]
          tunnel: w306 -> [w341 w345 w372]
          tunnel: [w341 w345 w372] -> w304
          frame "free running", Default {
            n153 = Bundle("tagged photons"=w342, "FFT modulous"=w343) -> (w344:T17)  [unwired: 1 in]
            n154 = Increment(x=w340) -> (x+1=w339:i32)
          }
          frame "run statistics" {
            n155 = call "GetHistogramFromXYgraph.vi"("Numeric"=w352, "image  IN"=w350, "Statistics (n-1)"=w351) -> ("Statistics (n)"=w349:cluster{dbl[][], dbl[][]})  [unwired: 8 in]
            n156 = case shown="2" "statistics show" {
              tunnel: w349 -> [w354 w359 w366]
              tunnel: [w353 w357 w360] -> w348
              frame 0, Default {
                n157 = Unbundle(w354) -> (w353:dbl[][])  [unwired: 1 out]
              }
              frame 1 {
                n158 = Unbundle(w359) -> (w358:dbl[][], w355:dbl[][])
                n159 = Square(x=w358) -> (x^2=w356:dbl[][])
                n160 = Subtract(x=w355, y=w356) -> (x-y=w357:dbl[][])
              }
              frame 2 {
                n161 = Unbundle(w366) -> (w362:dbl[][], w364:dbl[][])
                n162 = Square(x=w362) -> (x^2=w365:dbl[][])
                n163 = Subtract(x=w364, y=w365) -> (x-y=w363:dbl[][])
                n164 = Square Root(x=w363) -> (sqrt(x)=w361:dbl[][])
                n165 = Divide(x=w362, y=w361) -> (x/y=w360:dbl[][])
              }
            }
            "filtered  averaged" <- w348
            n166 = Increment(x=w352) -> (x+1=w346:i32)
            "current averaging" <- w352
          }
          frame "sequence recording" {
            n167 = local read "N current shoot"() -> (w368:i32)
            n168 = property on="sequence list" class="MCListbox (strict)"() -> ("Value"=w376:i32[])  [unwired: 2 in, 2 out]
            n169 = property on="sequence cluster" class="Clust (strict)"() -> ("Value"=w374:T5)  [unwired: 2 in, 2 out]
            n170 = property on="Current scan Tag" class="DigNum (strict)"() -> ("Value"=w367:i32)  [unwired: 2 in, 2 out]
            n171 = property on="result array" class="Arr (strict)"() -> ("Value"=w369:dbl[][])  [unwired: 2 in, 2 out]
            n172 = Increment(x=w368) -> (x+1=w378:i32)
            n173 = Insert Into Array(array=w376, index=w368, new element=w368) -> (w375:i32[])
            n174 = Replace Array Subset(array=w369, new element=w371, index (row)=w368, index (col)=w367) -> (w370:dbl[][])
            n175 = Unbundle By Name(w374) -> ("Nevent"=w377:i32)
            n176 = property on="sequence list" class="MCListbox (strict)"("Value"=w375) -> ()  [unwired: 2 in, 2 out]
            n177 = local write "N current shoot"(w378) -> ()
            n178 = property on="result array" class="Arr (strict)"("Value"=w370) -> ()  [unwired: 2 in, 2 out]
            n179 = Greater Or Equal?(x=w378, y=w377) -> (x >= y?=w379:bool)
            n180 = case shown="True" w379 {
              frame False {
              }
              frame True {
                n181 = property on="start sequence" class="Bool (strict)"("Value"=FALSE ("start sequence")) -> ()  [unwired: 2 in, 2 out]
                n182 = property on="loop state" class="Enum (strict)"("Value"=StateMachine."free running" ("loop state")) -> ()  [unwired: 2 in, 2 out]
              }
            }
          }
        }
        n183 = case shown="True" "Save all raw images" {
          tunnel: w303 -> [w331 w336]
          tunnel: w304 -> [_ w337]
          tunnel: [w330 w336] -> w302
          frame False {
            n184 = property on="loop state" class="Enum (strict)"() -> ("Value"=w332:T1)  [unwired: 2 in, 2 out]
            n185 = case shown="\"free running\", Default" w332 {
              tunnel: w331 -> [_ w334 w335]
              tunnel: [0 ("N current shoot") w334 w335] -> w330
              frame "free running", Default {
              }
              frame "run statistics" {
              }
              frame "sequence recording" {
              }
            }
          }
          frame True {
            n186 = call "SaveArrayAsTiff.vi"("name"="saving name", "Image Pixels (Float)"=w337, "number"=w336) -> ()  [unwired: 9 in]
          }
        }
      }
    }
    n187 = event shown="[0] Timeout" {
      selector: _ -> [_ _ _ _ _]
      dyn-events: _ -> [_ _ _ _ _]
      timeout: 0 -> [_ _ _ _ _]
      tunnel: [_ TRUE _ _ _] -> w297
      tunnel: [w391 w393 1 w412 w415] -> w285
      tunnel: w283 -> [w391 w393 _ w412 w415]
      tunnel: w282 -> [w390 w392 w396 w413 w414]
      tunnel: [w390 w392 w395 w413 w414] -> w281
      event Timeout {
        n188 = event-data() -> ()  [unwired: 1 in, 3 out]
        n189 = property on="fft cluster" class="Clust (strict)"() -> ("Value"=w384:T6)  [unwired: 2 in, 2 out]
        n190 = local read "Phase array"() -> (w385:dbl[])
        n191 = property on="result array" class="Arr (strict)"() -> ("Value"=w383:dbl[][])  [unwired: 2 in, 2 out]
        n192 = local read "sequence NbXZ"() -> (w388:dbl[][])
        n193 = call "unwrapFFT.vi"("phase offset"="phase offset", "active col"="active col", "sequence NBXZ"=w388, "phase array"=w385, "fft cluster"=w384, "result array IN"=w383) -> ("Intensity Graph"=w389:dbl[][], "FFT array"=w387:dbl[][])  [unwired: 4 in]
        n194 = property on="reconstructed image" class="IntGraph (strict)"("Value"=w389) -> ()  [unwired: 2 in, 2 out]
        n195 = property on="FFT acquire Graph" class="IntGraph (strict)"("Value"=w387) -> ()  [unwired: 2 in, 2 out]
      }
      event "Stop Button": Value Change {
        n196 = event-data() -> ()  [unwired: 1 in, 3 out]
      }
      event "run statistics": Value Change {
        n197 = event-data() -> ("NewVal"=w398:bool)  [unwired: 1 in, 5 out]
        n198 = case shown="True" w398 {
          tunnel: w396 -> [w399 w408]
          tunnel: [w399 w401] -> w395
          frame False {
            n199 = property on="loop state" class="Enum (strict)"("Value"=StateMachine."free running" ("loop state")) -> ()  [unwired: 2 in, 2 out]
          }
          frame True {
            n200 = Unbundle(w408) -> ("tagged photons"=w407:dbl[][], "FFT modulous"=w405:dbl[][])
            n201 = Multiply(x=0.0, y=w407) -> (x*y=w402:dbl[][])
            n202 = Multiply(x=w405, y=0.0) -> (x*y=w403:dbl[][])
            n203 = property on="loop state" class="Enum (strict)"("Value"=StateMachine."run statistics" ("loop state")) -> ()  [unwired: 2 in, 2 out]
            n204 = Bundle(w402, w403) -> (w401:cluster{dbl[][], dbl[][]})  [unwired: 1 in]
          }
        }
      }
      event "save scan": Value Change {
        n205 = event-data() -> ()  [unwired: 1 in, 6 out]
        n206 = property on="result array" class="Arr (strict)"() -> ("Value"=w411:dbl[][])  [unwired: 2 in, 2 out]
        n207 = call "SaveArray.vi"("name or relative path"="scan name", "array"=w411) -> ()  [unwired: 9 in, 1 out]
      }
      event "save noise": Value Change {
        n208 = event-data() -> ()  [unwired: 1 in, 6 out]
      }
    }
  }
  n209 = node-c288(w14) -> ()  [unwired: 1 out]
  n210 = flat-sequence {
    tunnel: w19 -> [_]
    tunnel: w18 -> [w420]
    tunnel: w16 -> [w419]
    frame #0 {
      n211 = invoke class="IICImagingControl" method="LiveStop"(reference=w419) -> (reference out=w418:refnum<k7>)  [unwired: 2 in, 2 out]
      n212 = property on="run statistics" class="Bool (strict)"("Value"=FALSE ("run statistics")) -> ()  [unwired: 2 in, 2 out]
      n213 = Release Queue(queue=w420) -> ()  [unwired: 2 in, 3 out]
      n214 = property on="live" class="Bool (strict)"("Value"=FALSE ("live")) -> ()  [unwired: 2 in, 2 out]
      n215 = call <userlib>:"IC_Clear.vi"("ICImagingControl 2"=w418) -> ()  [unwired: 1 out]
    }
  }
